vi "Load Final Data.vi"(11 "measured data":dbl[][](array[numeric])) -> ()   [LabVIEW 2015]
uses:
  Globals.vi
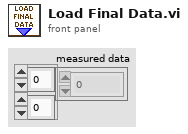
[diagram p1: front panel]
types:
  T1 = cluster{"x shift":dbl, "y shift":dbl, "z shift":dbl, "Theta x":dbl, "Theta y":dbl}
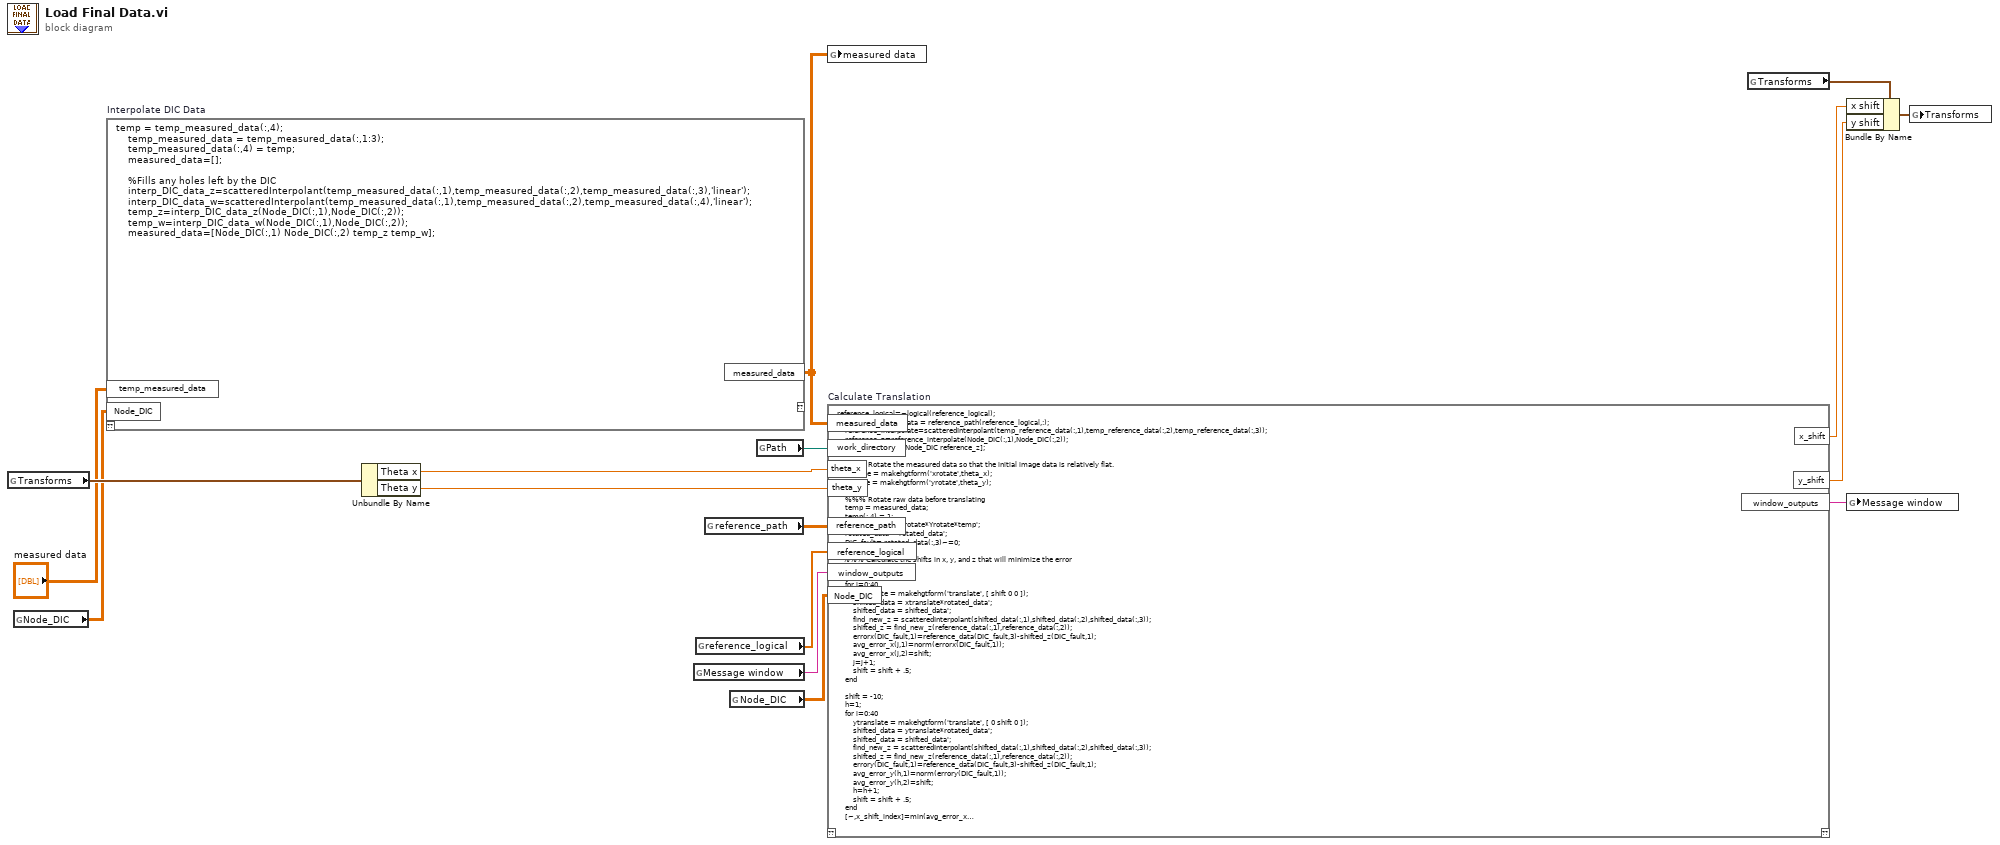
[diagram p0: block diagram]
diagram:
  n1 = global read "Globals.vi" "Transforms"() -> (w5:T1)
  n2 = global read "Globals.vi" "Node_DIC"() -> (w2:dbl[][])
  n3 = script code="temp = temp_measured_data(:,4);\n    temp_measured_data = temp_measured_data(:,1:3);\n    temp_measured_data(:,4) = temp;\n    measured_data=[];\n  \n    %Fills any holes left by the DIC\n    interp_DIC_data_z=scatteredInterpolant(temp_measured_data(:,1),temp_measured_data(:,2),temp_measured_data(:,3),'linear');\n    interp_DIC_data_w=scatteredInterpolant(temp_measured_data(:,1),temp_measured_data(:,2),temp_measured_data(:,4),'linear');\n    temp_z=interp_DIC_data_z(Node_DIC(:,1),Node_DIC(:,2));\n    temp_w=interp_DIC_data_w(Node_DIC(:,1),Node_DIC(:,2));\n    measured_data=[Node_DIC(:,1) Node_DIC(:,2) temp_z temp_w];" "Interpolate DIC Data"("temp_measured_data"="measured data", "Node_DIC"=w2) -> ("measured_data"=w3:dbl[][])  [unwired: 1 in, 1 out]
  n4 = Unbundle By Name(w5) -> ("Theta x"=w6:dbl, "Theta y"=w7:dbl)
  n5 = global read "Globals.vi" "Message window"() -> (w10:string)
  n6 = global read "Globals.vi" "reference_logical"() -> (w9:dbl[])
  n7 = global read "Globals.vi" "reference_path"() -> (w8:dbl[][])
  n8 = global read "Globals.vi" "Node_DIC"() -> (w11:dbl[][])
  n9 = global read "Globals.vi" "Path"() -> (w4:path)
  n10 = global write "Globals.vi" "measured data"(w3) -> ()
  n11 = script code="reference_logical=~logical(reference_logical);\n    temp_reference_data = reference_path(reference_logical,:);\n    reference_interpolate=scatteredInterpolant(temp_reference_data(:,1),temp_reference_data(:,2),temp_reference_data(:,3));\n    reference_z=reference_interpolate(Node_DIC(:,1),Node_DIC(:,2));\n    reference_data=[Node_DIC reference_z];\n    \n    %%% Rotate the measured data so that the initial image data is relatively flat.\n    Xrotate = makehgtform('xrotate',theta_x);\n    Yrotate = makehgtform('yrotate',theta_y);\n    \n    %%% Rotate raw data before translating\n    temp = measured_data;\n    temp(:,4) = 1;\n    rotated_data = Xrotate*Yrotate*temp';\n    rotated_data = rotated_data';\n    DIC_fault= rotated_data(:,3)~=0;\n    \n   %%% Calculate the shifts in x, y, and z that will minimize the error \n    j=1;\n    shift = -10;\n    for i=0:40\n        xtranslate = makehgtform('translate', [ shift 0 0 ]);\n        shifted_data = xtranslate*rotated_data';\n        shifted_data = shifted_data';\n        find_new_z = scatteredInterpolant(shifted_data(:,1),shifted_data(:,2),shifted_data(:,3));\n        shifted_z = find_new_z(reference_data(:,1),reference_data(:,2));\n        errorx(DIC_fault,1)=reference_data(DIC_fault,3)-shifted_z(DIC_fault,1);\n        avg_error_x(j,1)=norm(errorx(DIC_fault,1));\n        avg_error_x(j,2)=shift;\n        j=j+1;\n        shift = shift + .5;\n    end\n\n    shift = -10;\n    h=1;\n    for i=0:40\n        ytranslate = makehgtform('translate', [ 0 shift 0 ]);\n        shifted_data = ytranslate*rotated_data';\n        shifted_data = shifted_data';\n        find_new_z = scatteredInterpolant(shifted_data(:,1),shifted_data(:,2),shifted_data(:,3));\n        shifted_z = find_new_z(reference_data(:,1),reference_data(:,2));\n        errory(DIC_fault,1)=reference_data(DIC_fault,3)-shifted_z(DIC_fault,1);\n        avg_error_y(h,1)=norm(errory(DIC_fault,1));\n        avg_error_y(h,2)=shift;\n        h=h+1;\n        shift = shift + .5;\n    end\n    [~,x_shift_index]=min(avg_error_x(:,1));\n    [~,y_shift_index]=min(avg_error_y(:,1));\n    \n    x_shift = avg_error_x(x_shift_index,2);\n    y_shift = avg_error_y(y_shift_index,2);\n    \n    %________________________________________________________________________________________________\n    %Checks to see if the sheet has been formed\n    flat_check_x=max(avg_error_x(:,1))-min(avg_error_x(:,1));\n    flat_check_y=max(avg_error_y(:,1))-min(avg_error_y(:,1));\n    if flat_check_x<10\n        x_shift=0;\n    end\n    if flat_check_y<10\n       y_shift=0;\n    end\n    %________________________________________________________________________________________________\n    \n    figure(6);\n    plot(avg_error_x(:,2),avg_error_x(:,1));\n    hold on;\n    plot(avg_error_y(:,2),avg_error_y(:,1));\n    scatter(x_shift,avg_error_x(x_shift_index,1),'k');\n    scatter(y_shift,avg_error_y(y_shift_index,1),'r');\n    hold off;\n    legend('Error Magnitude X','Error Magnitude Y',strcat('Minimum X: ',num2str(x_shift)),strcat('Minimum Y: ',num2str(y_shift)));\n    xlabel('Translation (mm)');\n    ylabel('Magnitude of Error (mm)');\n    title('Average Error Magnitude vs Translation');\n    savefig(fullfile(work_directory,'Average Error Magnitude vs Translation.fig'));\n    fig_string = strcat(datestr(datetime('now')), '      Minimize Error Figure stored:  ', work_directory);\n    window_outputs = [window_outputs, newline, fig_string];\n    \n    % Write Transformation information to a text file\n    fileID = fopen(fullfile(work_directory,'Transformation Information.txt'),'w');\n    fprintf(fileID,'Transformation Information \\n');\n    fprintf(fileID,'Translation in x (mm): %4.3f\\n',x_shift);\n    fprintf(fileID,'Translation in y (mm): %4.3f\\n',y_shift);\n    fprintf(fileID,'Translation in z (mm): %4.3f\\n',z_shift);\n    fprintf(fileID,'Theta about x-axis (degrees): %4.3f\\n',theta_x);\n    fprintf(fileID,'Theta about y-axis (degrees): %4.3f\\n',theta_y);\n    fclose(fileID);\n    tran_string = strcat(datestr(datetime('now')), '      Transformation Information .txt file stored:  ', work_directory);\n    window_outputs = [window_outputs, newline, tran_string];\n    \n    % Output line divider\n    window_outputs = [window_outputs, newline, ' ----------- ', newline];" "Calculate Translation"("measured_data"=w3, "work_directory"=w4, "theta_x"=w6, "theta_y"=w7, "reference_path"=w8, "reference_logical"=w9, "window_outputs"=w10, "Node_DIC"=w11) -> ("y_shift"=w13:dbl, "x_shift"=w12:dbl, "window_outputs"=w16:string)  [unwired: 1 in, 1 out]
  n12 = global read "Globals.vi" "Transforms"() -> (w14:T1)
  n13 = Bundle By Name(cluster=w14, "x shift"=w12, "y shift"=w13) -> (w15:T1)
  n14 = global write "Globals.vi" "Message window"(w16) -> ()
  n15 = global write "Globals.vi" "Transforms"(w15) -> ()
